vi "StartSequenceAcq.vi"(8 "error in (no error)":errorcluster, 11 "ImagingMode in":refnum<class "ImagingMode.lvclass">) -> (0 "error out":errorcluster, 3 "ImagingMode out":refnum<class "ImagingMode.lvclass">)   [LabVIEW 2020, in "ImagingMode.lvlib" / "ImagingMode.lvclass"]
uses:
  ImagingMode.lvclass
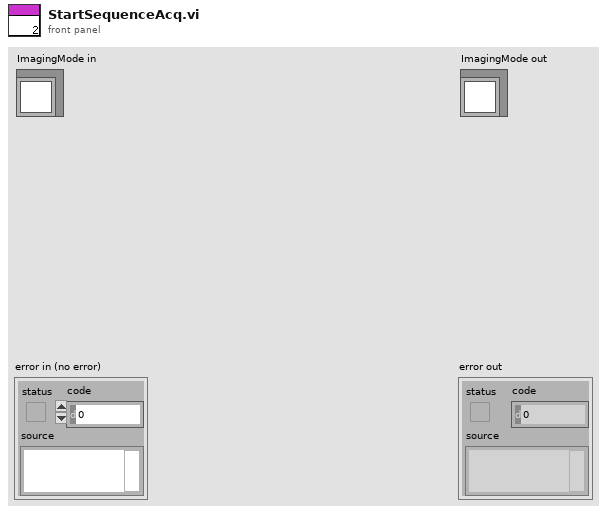
[diagram p1: front panel]
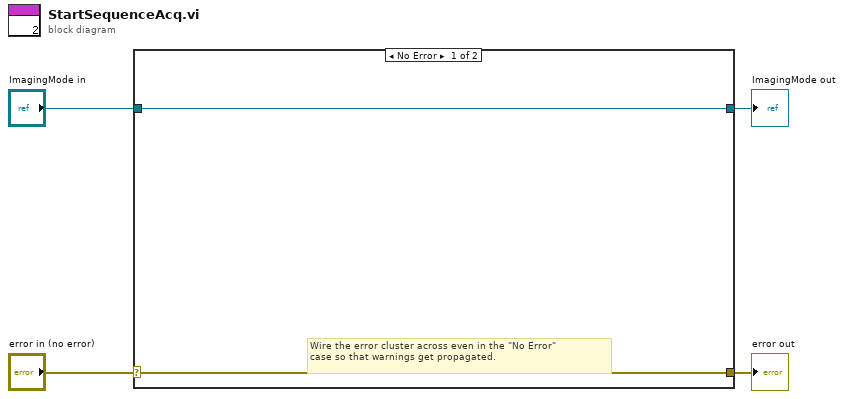
[diagram p0: block diagram]
diagram:
  n1 = case shown="No Error" "error in (no error)" {
    selector: "error in (no error)" -> [w5 w8]
    tunnel: [w5 w8] -> w3
    tunnel: [w6 w7] -> w1
    tunnel: "ImagingMode in" -> [w6 w7]
    frame No Error {
      # "Wire the error cluster across even in the \"No Error\"\ncase so that warnings get propagated."
    }
    frame Error {
    }
  }
  "error out" <- w3
  "ImagingMode out" <- w1
